vi "Read Sonar Test.vi"() -> ()   [LabVIEW 2016]
panel:
  in  "x":dbl
  out "Distance 2":dbl
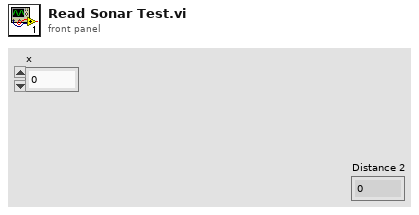
[diagram p1: front panel]
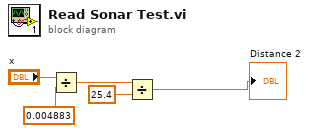
[diagram p0: block diagram]
diagram:
  n1 = Divide(x="x", y=0.004883) -> (x/y=w4:dbl)
  n2 = Divide(x=w4, y=25.4) -> (x/y=→"Distance 2":dbl)
